vi "Config Process.vi"(8 "error in (no error)":errorcluster, 10 "Queues":T1, 11 "UE Data Container":T2) -> (0 "error out":errorcluster)   [LabVIEW 2017]
doc: "Interface to Config DB for Read/Search/Update records by the Controller.\n[Covers: CD5]"
uses:
  Shared Data/User Events/UE Data Container.ctl
  Shared Data/Queues/Controls/Queues.ctl
  Controller/Controls/UI CMD.ctl
  Controller/Controls/Controller CMD.ctl
  Error Handler/Controls/Error CMD.ctl
  Controls/Config CMD.ctl
  Controls/Config Array.ctl
  Controls/Config Data.ctl
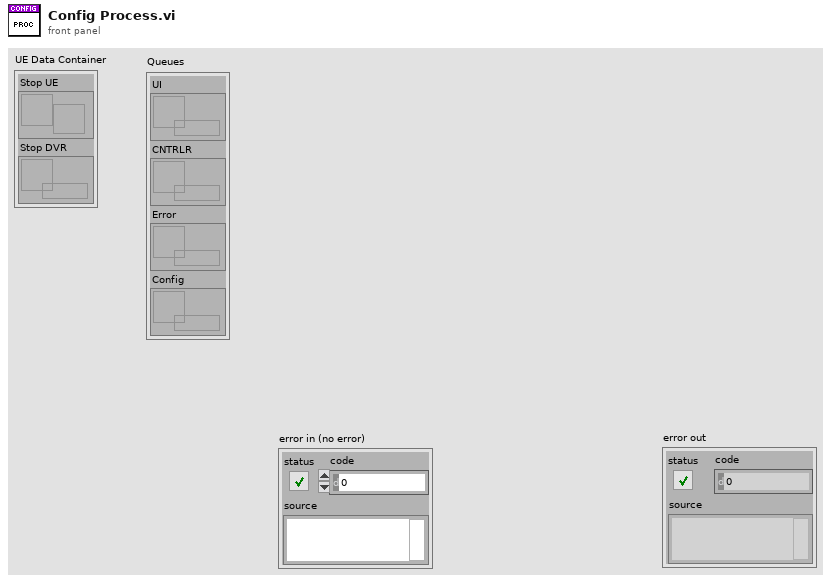
[diagram p1: front panel]
types:
  T1 = typedef "Queues.ctl" = cluster{"UI":refnum<queue>, "CNTRLR":refnum<queue>, "Error":refnum<queue>, "Config":refnum<queue>}
  T2 = typedef "UE Data Container.ctl" = cluster{"Stop UE":refnum<user-event>, "Stop DVR":refnum<data-value>}
  T3 = typedef "Config Array.ctl" = T4[]
  T4 = typedef "Config Data.ctl" = cluster{"Account Number":u32, "Last Name":string, "First Name":string, "Balance":dbl}
  T5 = typedef "Config CMD.ctl" = cluster{"CMD":enum16{"Idle", "Read", "Search", "Update", "Stop"}, "Data":variant}
  T6 = enum16{"Idle", "Read", "Search", "Update", "Stop"}
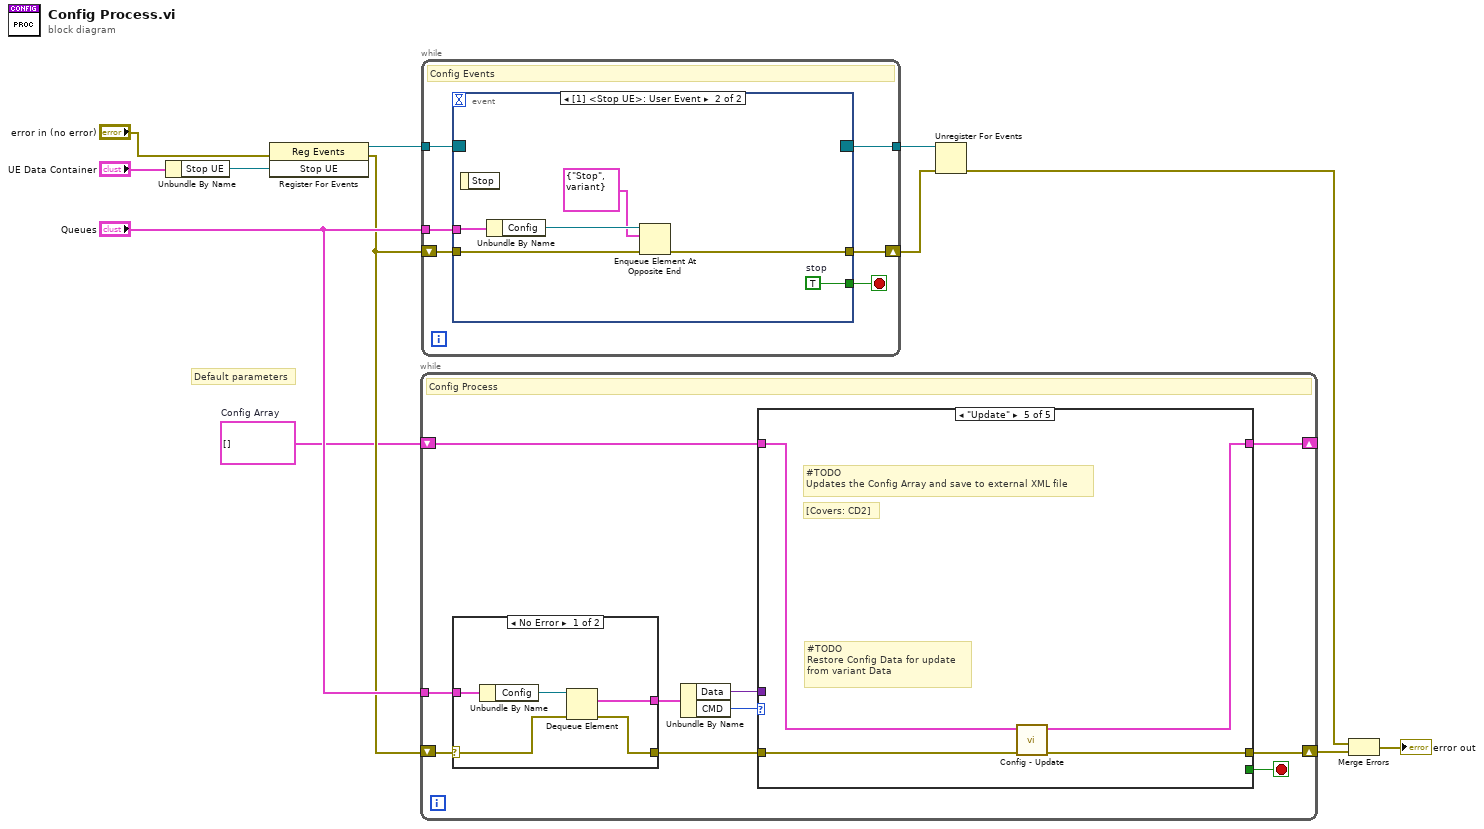
[diagram p0: block diagram]
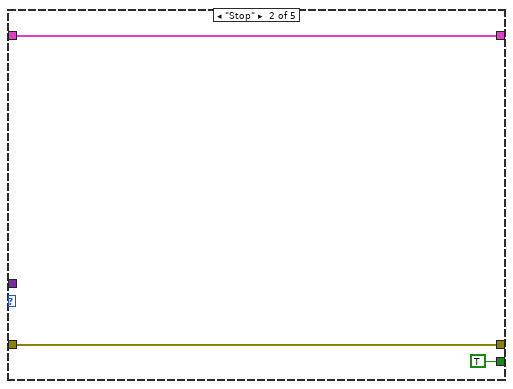
[diagram p3: hidden frame]
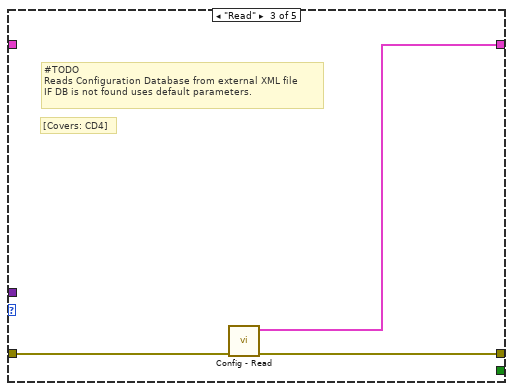
[diagram p4: hidden frame]
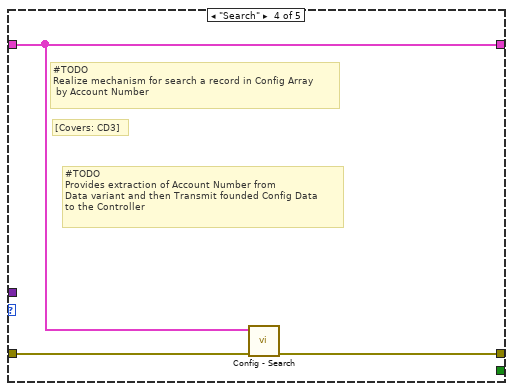
[diagram p5: hidden frame]
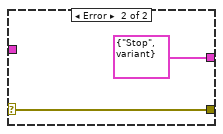
[diagram p6: hidden frame]
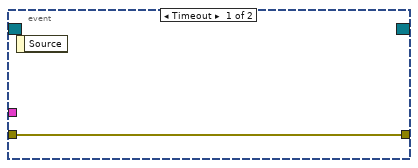
[diagram p7: hidden frame]
diagram:
  w1 = T3 []  # Config Array
  # "Default parameters"
  n1 = Unbundle By Name("UE Data Container") -> ("Stop UE"=w11:refnum<user-event>)
  n2 = register-events(error in="error in (no error)", w11) -> (reference out=w9:refnum<event-registration>, error out=w5:errorcluster)  [unwired: 1 in]
  n3 = while {
    tunnel: "Queues" -> [w22]
    shift-right: [w16] -> w4
    shift-left: w5 -> [w21]
    shift-right: [w13] -> _
    shift-left: w1 -> [w14]
    stop <- w15 stop-if-true
    # "Config Process"
    n4 = case shown="No Error" w21 {
      selector: w21 -> [w40 w43]
      tunnel: w22 -> [w42 _]
      tunnel: [w39 T5 {"CMD"=enum."Stop", "Data"=variant} ("Config CMD")] -> w20
      tunnel: [w38 w43] -> w17
      frame No Error {
        n5 = Unbundle By Name(w42) -> ("Config"=w41:refnum<queue>)
        n6 = Dequeue Element(queue=w41, error in (no error)=w40) -> (element=w39:T5, error out=w38:errorcluster)  [unwired: 1 in, 2 out]
      }
      frame Error {
      }
    }
    n7 = Unbundle By Name(w20) -> ("Data"=w18:variant, "CMD"=w19:T6)
    n8 = case shown="\"Update\"" w19 {
      tunnel: w18 -> [_ _ _ _ _]
      tunnel: w17 -> [w24 w27 w30 w33 w37]
      tunnel: [w24 w27 w29 w32 w36] -> w16
      tunnel: [_ TRUE _ _ _] -> w15
      tunnel: w14 -> [w23 w25 _ w31 w35]
      tunnel: [w23 w25 w28 w31 w34] -> w13
      frame "Idle", Default {
      }
      frame "Stop" {
      }
      frame "Read" {
        # "[Covers: CD4]"
        # "#TODO\nReads Configuration Database from external XML file\nIF DB is not found uses default parameters."
        n9 = call "Config - Read.vi"("error in (no error)"=w30) -> ("error out"=w29:errorcluster, "Config Array"=w28:T3)  [unwired: 9 in]
      }
      frame "Search" {
        # "#TODO\nProvides extraction of Account Number from\nData variant and then Transmit founded Config Data\nto the Controller"
        # "[Covers: CD3]"
        # "#TODO\nRealize mechanism for search a record in Config Array\n by Account Number"
        n10 = call "Config - Search.vi"("error in (no error)"=w33, "Config Array"=w31) -> ("error out"=w32:errorcluster)  [unwired: 8 in, 1 out]
      }
      frame "Update" {
        # "#TODO\nRestore Config Data for update\nfrom variant Data"
        # "[Covers: CD2]"
        # "#TODO\nUpdates the Config Array and save to external XML file"
        n11 = call "Config - Update.vi"("error in (no error)"=w37, "Config Array"=w35) -> ("error out"=w36:errorcluster, "Config Array"=w34:T3)  [unwired: 8 in]
      }
    }
  }
  n12 = while {
    tunnel: w9 -> [w50]
    tunnel: [w49] -> w8
    tunnel: "Queues" -> [w47]
    shift-right: [w45] -> w7
    shift-left: w5 -> [w46]
    stop <- w48 stop-if-true
    # "Config Events"
    n13 = event shown="[1] <Stop UE>: User Event" {
      selector: w50 -> [_ _]
      dyn-events: [_ _] -> w49
      timeout: _ -> [_ _]
      tunnel: [_ w57] -> w48
      tunnel: w47 -> [_ w56]
      tunnel: w46 -> [w51 w54]
      tunnel: [w51 w53] -> w45
      event Timeout {
        n14 = event-data() -> ()  [unwired: 1 in, 1 out]
      }
      event User Event {
        w57 = TRUE  # stop
        n15 = event-data() -> ()  [unwired: 1 in, 1 out]
        n16 = Unbundle By Name(w56) -> ("Config"=w55:refnum<queue>)
        n17 = Enqueue Element At Opposite End(queue=w55, element=T5 {"CMD"=enum."Stop", "Data"=variant} ("Config CMD"), error in (no error)=w54) -> (error out=w53:errorcluster)  [unwired: 1 in, 2 out]
      }
    }
  }
  n18 = Unregister For Events(event registration refnum=w8, error in=w7) -> (error out=w3:errorcluster)
  n19 = Merge Errors(w3, w4) -> (→"error out":errorcluster)
